vi "Merge Error.vi"(10 "Error":errorcluster) -> (2 "Msg Strategy":refnum<class "Msg Strategy.lvclass">)   [LabVIEW 2021, in "Merge Error Msg Strategy.lvlib"]
uses:
  Merge Error Msg Strategy.lvlib
  jettl/Msg Strategy/Msg Strategy.lvclass
  Merge Error Msg Strategy/Merge Error Msg Strategy.lvclass
  C:/git/jettl/jettl/jettl/Msg Strategy/Msg Strategy.lvclass
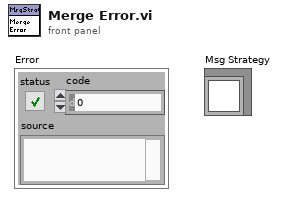
[diagram p1: front panel]
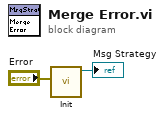
[diagram p0: block diagram]
diagram:
  n1 = call "Init.vi"("Error"="Error") -> ("Merge Error Msg Strategy out"=→"Msg Strategy":refnum<class "Merge Error Msg Strategy.lvclass">)  [unwired: 10 in]
